vi "FET_vs_GATE.vi"() -> ()   [LabVIEW 2014]
doc: "FET1 = I_DS vs V_DS\nMisura la caratteristica di un FET canale N\nfissando V sul DRAIN e variando V _GATE\nFM & ADL 2015/11"
uses:
  <vilib>/DAQmx/write.llb/DAQmx Write (Analog DBL 1Chan 1Samp).vi
  <vilib>/DAQmx/create/channels.llb/DAQmx Create Channel (AO-Voltage-Basic).vi
  <vilib>/DAQmx/configure/timing.llb/DAQmx Timing (Sample Clock).vi
  <vilib>/DAQmx/miscellaneous.llb/DAQmx Fill In Error Info.vi
  <vilib>/Utility/file.llb/Write To Spreadsheet File (DBL).vi
panel:
  in  "R_SOURCE (kOhm)":dbl=0.1 format="%_4g"
  in  "Vin_DRAIN":dbl=8.0 min=-10.0 max=10.0 step=0.025 format="%.3f"
  in  "Fondo Scala AI1":dbl(ring)=0.5 items=["10"=10.0, "5"=5.0, "0.5"=0.5, "0.05"=0.05]
  in  "SALVA I DATI":bool=TRUE caption="ON\nOFF"
  out "V_GATE":dbl=3.599954919857113 format="%_3g"
  out "No Misura":i32=50
  in  "Fondo Scala AI0":dbl(ring)=10.0 items=["10"=10.0, "5"=5.0, "0.5"=0.5, "0.05"=0.05]
  out "Corrente DRAIN-SOURCE in funzione della V_GS":cluster{dbl[], dbl[]}(graph)={[1.9981831321829053, 2.030191872969443, 2.0613994292865128, 2.0922082563331235, 2.1224908424441526, 2.1515260327676393, 2.1797801983407994, 2.2064965235119693, 2.2315412157189325, 2.255239850892698, 2.2771516312703755, 2.2978207685883314, 2.3169172499175352, 2.334543347737455, 2.3512081570563446, 2.3665449329182087, 2.380900124044754, 2.3944435512784312, 2.406974074357661, 2.4188575766566833, 2.4301048502434446, 2.440706999211377, 2.450855189249363, 2.4604511635026034, 2.4696220516734826, 2.478384474800423, 2.486738454629593, 2.494858755309532, 2.5026145218084723, 2.5099018840953446, 2.5170611413378854, 2.5239921430992713, 2.5306892328053556, 2.5371113090814252, 2.543399347912315, 2.5494290737894705, 2.5553619568366166, 2.5610709073752305, 2.5666229191022483, 2.571990527012361, 2.57718807867996, 2.5823530250154825, 2.5873612764256477, 2.592241404938716, 2.5970732082957206, 2.601467811295206, 2.60604363484835, 2.610603529114049, 2.614941762510598, 2.6204185206219806], [0.01609165966009779, 0.024248249561236203, 0.03624002118600659, 0.05381936354071554, 0.07887260394176762, 0.11314160015798944, 0.1592708954842394, 0.21916343445723901, 0.2930448034060055, 0.38369249277314205, 0.4889817452568651, 0.610701468621461, 0.7471076540084098, 0.8952075707673154, 1.0576194150977678, 1.2313201743182773, 1.4131805417063052, 1.6060699589704666, 1.8052551504654872, 2.013733234673289, 2.228491396426309, 2.4474497835401303, 2.673931459057007, 2.9053798858838378, 3.139043389899563, 3.379081878112971, 3.6202604156909395, 3.8674248678920633, 4.117674323469577, 4.368395013574554, 4.6243432631562325, 4.882521425775324, 5.141272381125395, 5.404132195228646, 5.666860158721173, 5.934067246550941, 6.202387281860366, 6.470468879634188, 6.742579417738825, 7.016165884999411, 7.288437880391723, 7.564243057766067, 7.839352658498882, 8.117905646009614, 8.397866838658972, 8.676102675297734, 8.957604840545619, 9.240189606750402, 9.521445248843875, 9.795363992351323]}
  out "V_SOURCE":dbl=0.9795363992351324 format="%_3f"
  in  "# misure":i16=50
  in  "Vmax":dbl=3.6 max=100000.0
  in  "Vmin":dbl=2.0
  # "Valore consigliato  R_SOURCE = 100 Ohm"
  # "1) Selezionare il valore minimo e massimo della tensione (Vin_GATE) applicata al GATE  ed il numero di valori (equispaziati  tra gli estremi). \nSelezionare la tensione fissa applicata al DRAIN.\nSelezionare il valore della resistenza in serie al SOURCE."
  # "2) Collegare il CB22 e CB68 al GATE,   \n    CB21 al DRAIN,  \n    CB33 alla resistenza in serie al SOURCE.\nLa terra del circuito DEVE essere in comune alla terra della scheda (CB29)."
  # "Durante la misura gli indicatori mostrano i valori di I_DRAIN,    V_GATE , V_SOURCE ed il numero progressivo della misura.\n\nSul grafico viene mostrata la corrente che scorre da DRAIN a SOURCE  in funzione della tensione GATE-SOURCE."
  # "NO\nSI"
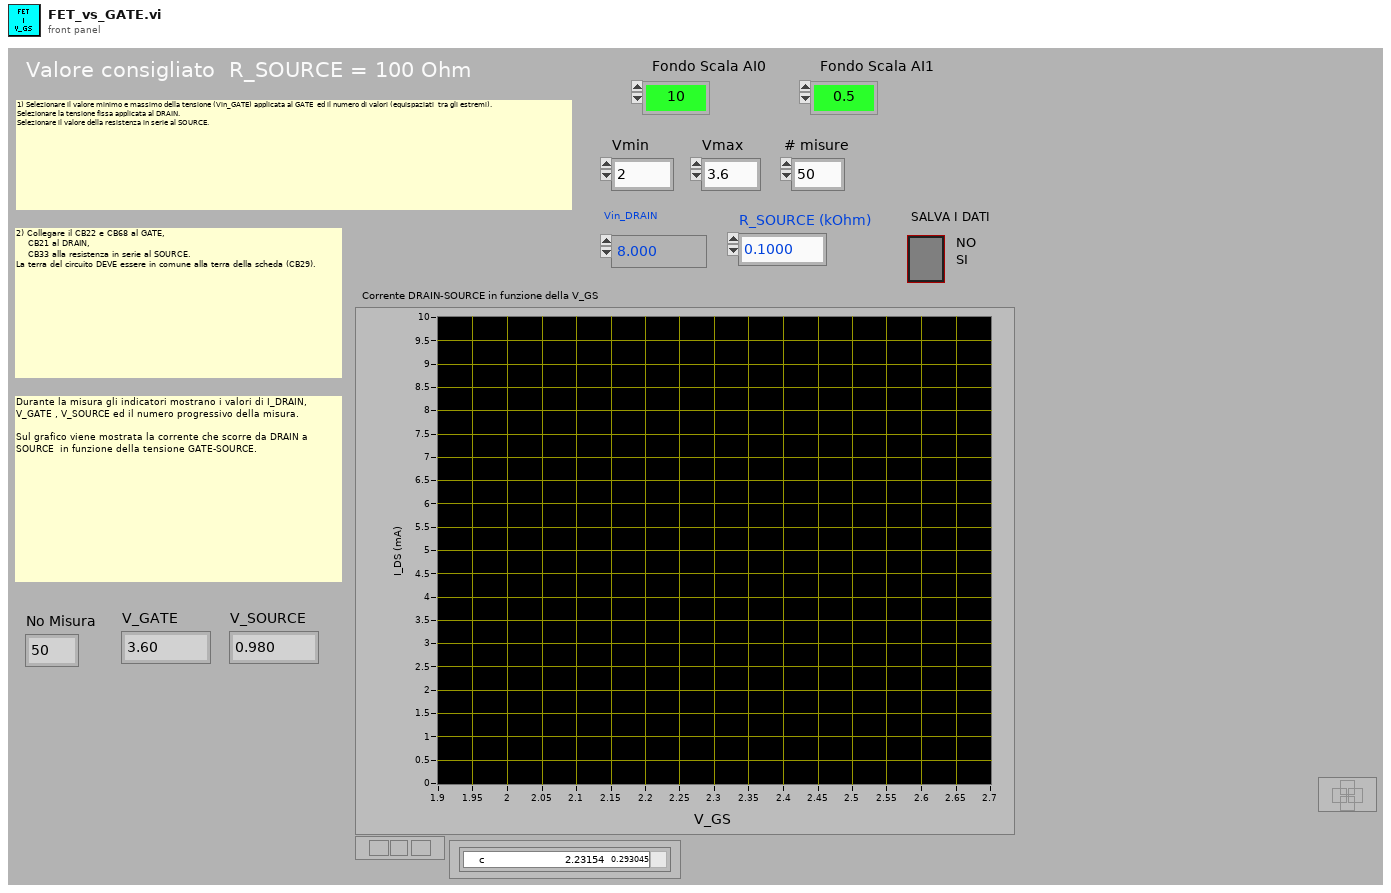
[diagram p1: front panel]
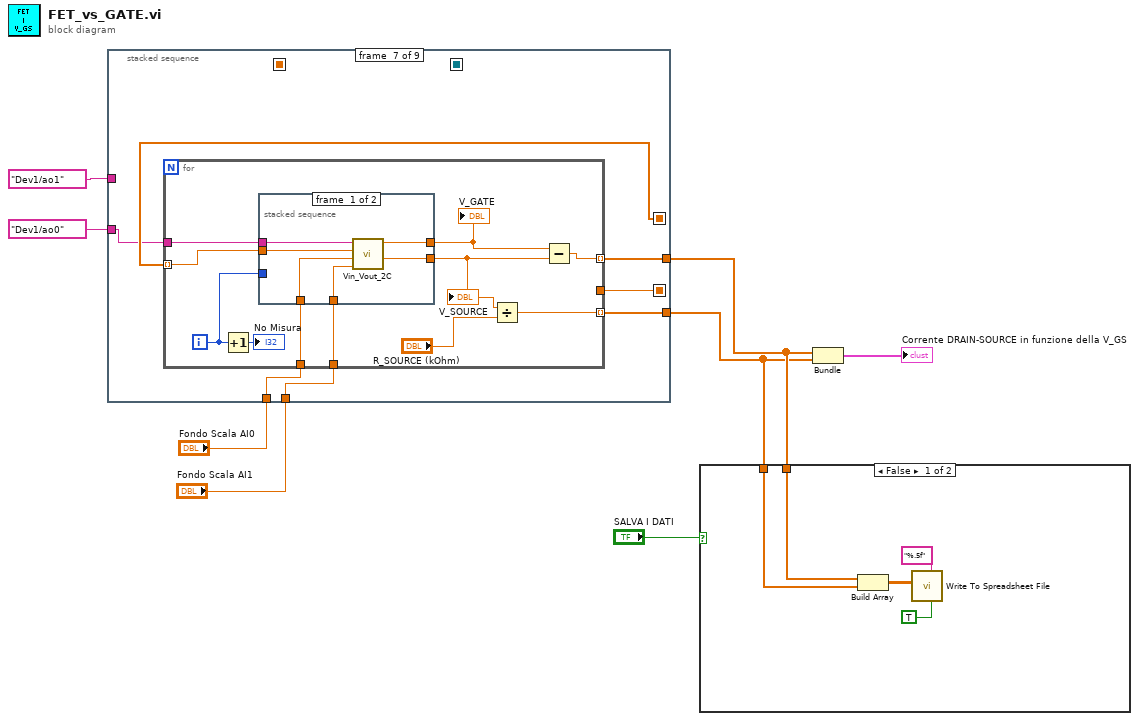
[diagram p0: block diagram]
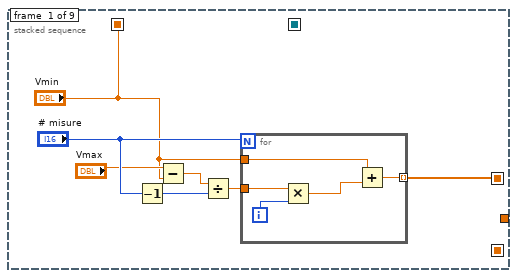
[diagram p3: hidden frame]
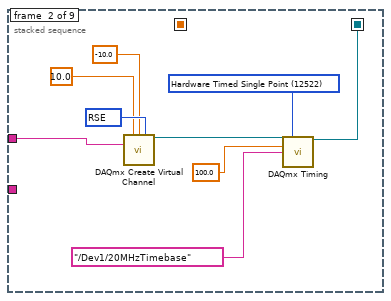
[diagram p4: hidden frame]
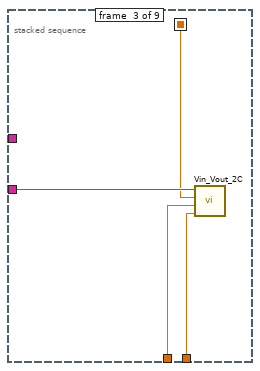
[diagram p5: hidden frame]
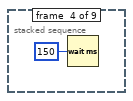
[diagram p6: hidden frame]
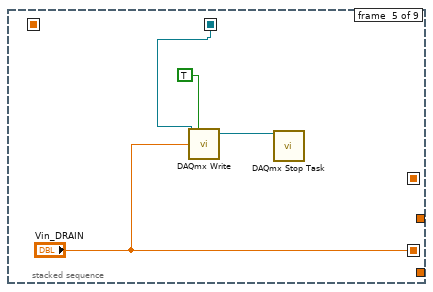
[diagram p7: hidden frame]
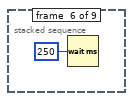
[diagram p8: hidden frame]
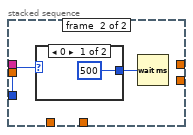
[diagram p9: hidden frame]
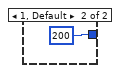
[diagram p10: hidden frame]
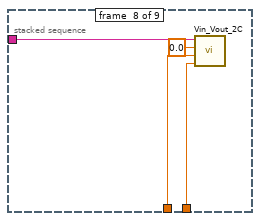
[diagram p11: hidden frame]
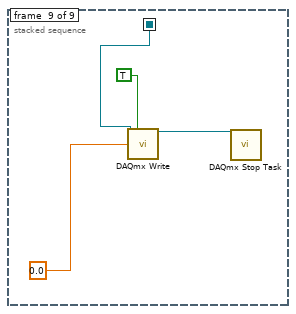
[diagram p12: hidden frame]
diagram:
  n1 = stacked-sequence {
    seq-local: [w12 _ _ _ _ _ _ _ _] -> [_ _ _ _ _ _ w45 _ _]
    seq-local: [_ w22 _ _ _ _ _ _ _] -> [_ _ _ _ w37 _ _ _ w74]
    seq-local: [_ _ _ _ "Vin_DRAIN" _ _ _ _] -> [_ _ _ _ _ _ w40 _ _]
    seq-local: ["Vmin" _ _ _ _ _ _ _ _] -> [_ _ w30 _ _ _ _ _ _]
    tunnel: "Fondo Scala AI1" -> [_ _ w31 _ _ _ w46 w69 _]
    tunnel: "Fondo Scala AI0" -> [_ _ w32 _ _ _ w44 w70 _]
    tunnel: tag "Dev1/ao1" ("physical channels") -> [_ w21 _ _ _ _ _ _ _]
    tunnel: tag "Dev1/ao0" ("physical channels") -> [_ _ w33 _ _ _ w43 w71 _]
    tunnel: [_ _ _ _ _ _ w42 _ _] -> w1
    tunnel: [_ _ _ _ _ _ w41 _ _] -> w2
    frame #0 {
      n2 = Decrement(x="# misure") -> (x-1=w14:i16)
      n3 = Subtract(x="Vmax", y="Vmin") -> (x-y=w15:dbl)
      n4 = Divide(x=w15, y=w14) -> (x/y=w13:dbl)
      n5 = for {
        N: "# misure" -> [_]
        tunnel: "Vmin" -> [w20]
        tunnel: [w19] -> w12 mode=indexing
        tunnel: w13 -> [w18]
        i -> [w17]
        n6 = Multiply(x=w18, y=w17) -> (x*y=w16:dbl)
        n7 = Add(x=w20, y=w16) -> (x+y=w19:dbl)
      }
    }
    frame #1 {
      w26 = 12522 items=["Finite Samples"=10178, "Continuous Samples"=10123, "Hardware Timed Single Point"=12522] ("sample mode")
      w29 = 10083 items=["Default"=-1, "RSE"=10083, "Differential"=10106, "Pseudodifferential"=12529] ("output terminal configuration")
      n8 = call-poly <vilib>:"DAQmx Create Virtual Channel.vi"("maximum value"=10.0, "minimum value"=-10.0, "output terminal configuration"=w29, "physical channels"=w21) -> ("task out"=w24:refnum<k21>)  [unwired: 5 in, 6 out]
      n9 = call-poly <vilib>:"DAQmx Timing.vi"("task/channels in"=w24, "sample mode"=w26, "rate"=100.0, "source"=tag "/Dev1/20MHzTimebase") -> ("task out"=w22:refnum<k21>)  [unwired: 3 in, 8 out]
    }
    frame #2 {
      n10 = call "Vin_Vout_2C.vi"("Fondo Scala AI1 (33)"=w31, "Fondo Scala AI0 (68)"=w32, "V in volt"=w30, "Canale uscita"=w33) -> ()  [unwired: 4 out]
    }
    frame #3 {
      n11 = Wait (ms)(milliseconds to wait=u32 150) -> ()  [unwired: 1 out]
    }
    frame #4 {
      n12 = call-poly <vilib>:"DAQmx Write.vi"("task/channels in"=w37, "auto start"=TRUE, "data"="Vin_DRAIN") -> ("task out"=w36:refnum<k21>)  [unwired: 1 in, 11 out]
      n13 = call <vilib>:"DAQmx Stop Task.vi"("task/channels in"=w36) -> ()  [unwired: 1 in, 14 out]
    }
    frame #5 {
      n14 = Wait (ms)(milliseconds to wait=u32 250) -> ()  [unwired: 1 out]
    }
    frame #6 {
      n15 = for {
        tunnel: w45 -> [w52] mode=indexing
        tunnel: w46 -> [w57]
        tunnel: w44 -> [w55]
        tunnel: w43 -> [w53]
        tunnel: [w47] -> w42 mode=indexing
        tunnel: [w51] -> w41 mode=indexing
        tunnel: w40 -> [_]
        i -> [w54]
        n16 = Increment(x=w54) -> (x+1=→"No Misura":i32)
        n17 = stacked-sequence {
          tunnel: w52 -> [w61 _]
          tunnel: w57 -> [w62 _]
          tunnel: w55 -> [w63 _]
          tunnel: w54 -> [_ w64]
          tunnel: w53 -> [w60 _]
          tunnel: [w59 _] -> w50
          tunnel: [w58 _] -> w49
          frame #0 {
            n18 = call "Vin_Vout_2C.vi"("Fondo Scala AI1 (33)"=w62, "Fondo Scala AI0 (68)"=w63, "V in volt"=w61, "Canale uscita"=w60) -> ("V1 medio"=w58:dbl, "V0 medio"=w59:dbl)  [unwired: 2 out]
          }
          frame #1 {
            n19 = case shown="0" w64 {
              tunnel: [500 u32 200 ("milliseconds to wait")] -> w65
              frame 0 {
              }
              frame 1, Default {
              }
            }
            n20 = Wait (ms)(milliseconds to wait=w65) -> ()  [unwired: 1 out]
          }
        }
        "V_SOURCE" <- w49
        "V_GATE" <- w50
        n21 = Divide(x=w49, y="R_SOURCE (kOhm)") -> (x/y=w47:dbl)
        n22 = Subtract(x=w50, y=w49) -> (x-y=w51:dbl)
      }
    }
    frame #7 {
      n23 = call "Vin_Vout_2C.vi"("Fondo Scala AI1 (33)"=w69, "Fondo Scala AI0 (68)"=w70, "V in volt"=0.0, "Canale uscita"=w71) -> ()  [unwired: 4 out]
    }
    frame #8 {
      n24 = call-poly <vilib>:"DAQmx Write.vi"("task/channels in"=w74, "auto start"=TRUE, "data"=0.0) -> ("task out"=w72:refnum<k21>)  [unwired: 1 in, 11 out]
      n25 = call <vilib>:"DAQmx Stop Task.vi"("task/channels in"=w72) -> ()  [unwired: 1 in, 14 out]
    }
  }
  n26 = case shown="False" "SALVA I DATI" {
    tunnel: w2 -> [w80 _]
    tunnel: w1 -> [w79 _]
    frame False {
      n27 = Build Array(w80, w79) -> (w76:dbl[][])
      n28 = call-poly <vilib>:"Write To Spreadsheet File.vi"("transpose? (no:F)"=TRUE, "format (%.3f)"="%.5f", "2D data"=w76) -> ()  [unwired: 3 in, 3 out]
    }
    frame True {
    }
  }
  n29 = Bundle(w2, w1) -> (→"Corrente DRAIN-SOURCE in funzione della V_GS":cluster{dbl[], dbl[]})  [unwired: 1 out]
